vi "Platform 송신 Stop.vi"() -> ()   [LabVIEW 2016]
panel:
  in  "Platform 송신 Stop":bool
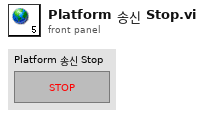
[diagram p1: front panel]
diagram:
